vi "Update version.vi"(6 "Top Level/Always Included VIs":path[](array[path]), 7 "Main Destination Path":path, 9 "Target Name":string, 10 "Build Specification Name":string, 11 "Project Path":path) -> (0 "error out":errorcluster)   [LabVIEW 2016]
uses:
  <vilib>/AppBuilder/AB_API_Simple/Get Build Specification Version (path).vi
  <vilib>/AppBuilder/AB_API_Simple/NI_App_Builder_API.lvlib
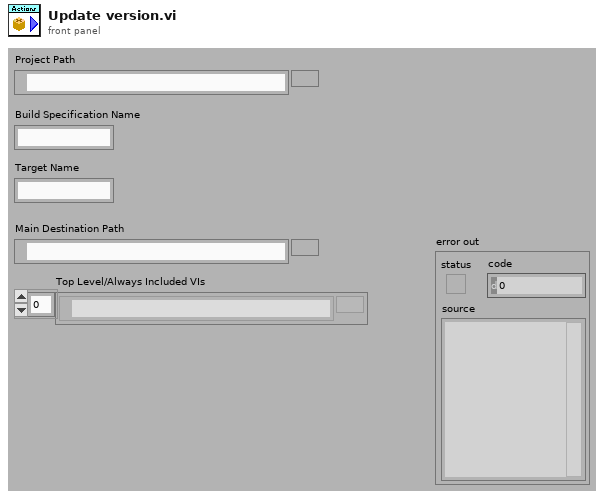
[diagram p1: front panel]
types:
  T1 = typedef "NI_App_Builder_API.lvlib/Build Specification Version.ctl" = cluster{"Major":u16, "Minor":u16, "Fix":u16, "Build":u16}
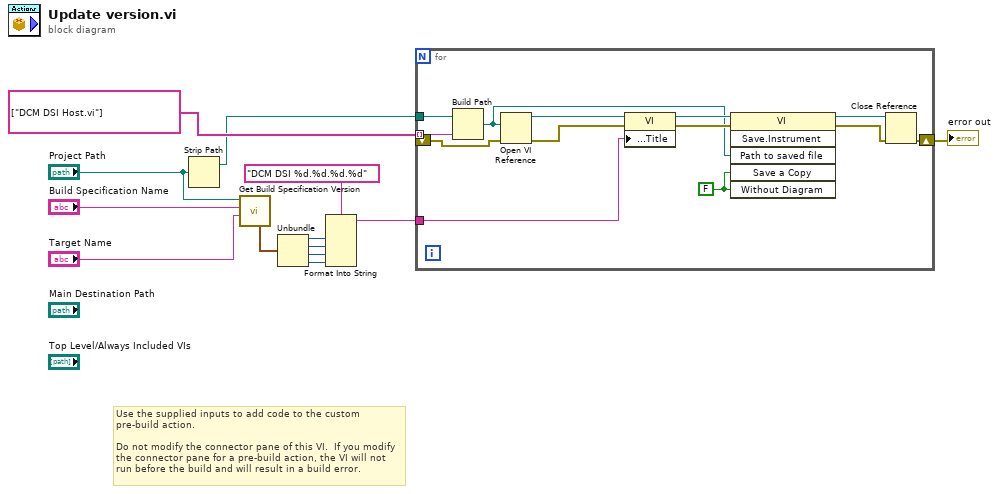
[diagram p0: block diagram]
diagram:
  # "Use the supplied inputs to add code to the custom pre-build action.\n\nDo not modify the connector pane of this VI.  If you modify the connector pane for a pre-build action, the VI will not run before the build and will result in a build error."
  n1 = Strip Path(path="Project Path") -> (stripped path=w1:path)  [unwired: 1 out]
  n2 = call-poly <vilib>:"Get Build Specification Version.vi"("Name of target (My Computer)"="Target Name", "Name of build specification"="Build Specification Name", "Path to project"="Project Path") -> ("Build Specification Version"=w10:T1)  [unwired: 7 in, 1 out]
  n3 = Unbundle(w10) -> ("Major"=w9:u16, "Minor"=w8:u16, "Fix"=w7:u16, "Build"=w6:u16)
  n4 = Format Into String(format string="DCM DSI %d.%d.%d.%d", w9, w8, w7, w6) -> (resulting string=w4:string)  [unwired: 2 in, 1 out]
  n5 = for {
    tunnel: string[] ["DCM DSI Host.vi"] ("name or relative path") -> [w26] mode=indexing
    tunnel: w4 -> [w24]
    tunnel: w1 -> [w17]
    shift-right: [w23] -> w3
    shift-left: _ -> [w14]
    w16 = FALSE ("Without Diagram")
    n6 = Build Path(base path=w17, name or relative path=w26) -> (appended path=w15:path)
    n7 = Open VI Reference(vi path=w15, error in (no error)=w14) -> (vi reference=w25:refnum<vi>, error out=w22:errorcluster)  [unwired: 4 in]
    n8 = property class="VI"(reference=w25, error in=w22, "Front Panel.Title"=w24) -> (reference out=w21:refnum<vi>, error out=w20:errorcluster)
    n9 = invoke class="VI" method="Save.Instrument"(reference=w21, error in=w20, "Path to saved file"=w15, "Save a Copy"=w16, "Without Diagram"=w16) -> (reference out=w18:refnum<vi>, error out=w19:errorcluster)  [unwired: 1 in, 4 out]
    n10 = Close Reference(reference=w18, error in (no error)=w19) -> (error out=w23:errorcluster)
  }
  "error out" <- w3
